vi "3D-10点建面算高度.vi"(9 "布尔":bool, 10 "Max 位置数组":cluster{"列":dbl, "行":dbl, "Z":dbl}[](array[cluster]), 11 "基准点数组":cluster{"列":dbl, "行":dbl, "Z":dbl}[](array[cluster])) -> (0 "Z":string[](array[string]), 1 "Result":string, 3 "Z轴相对高度":dbl[](array[numeric])=[0.07904724866187265, 0.12091362208012832, 0.13921122232312513, 0.04880031245592914, 1.3322676295365137e-15, 0.021807097148537454, 1.9984014443047706e-15, 0.020027978783221875, 0.014032416135081075, -0.06192666880740527, -0.09122658763869643, -3.663735981225413e-15])   [LabVIEW 2015]
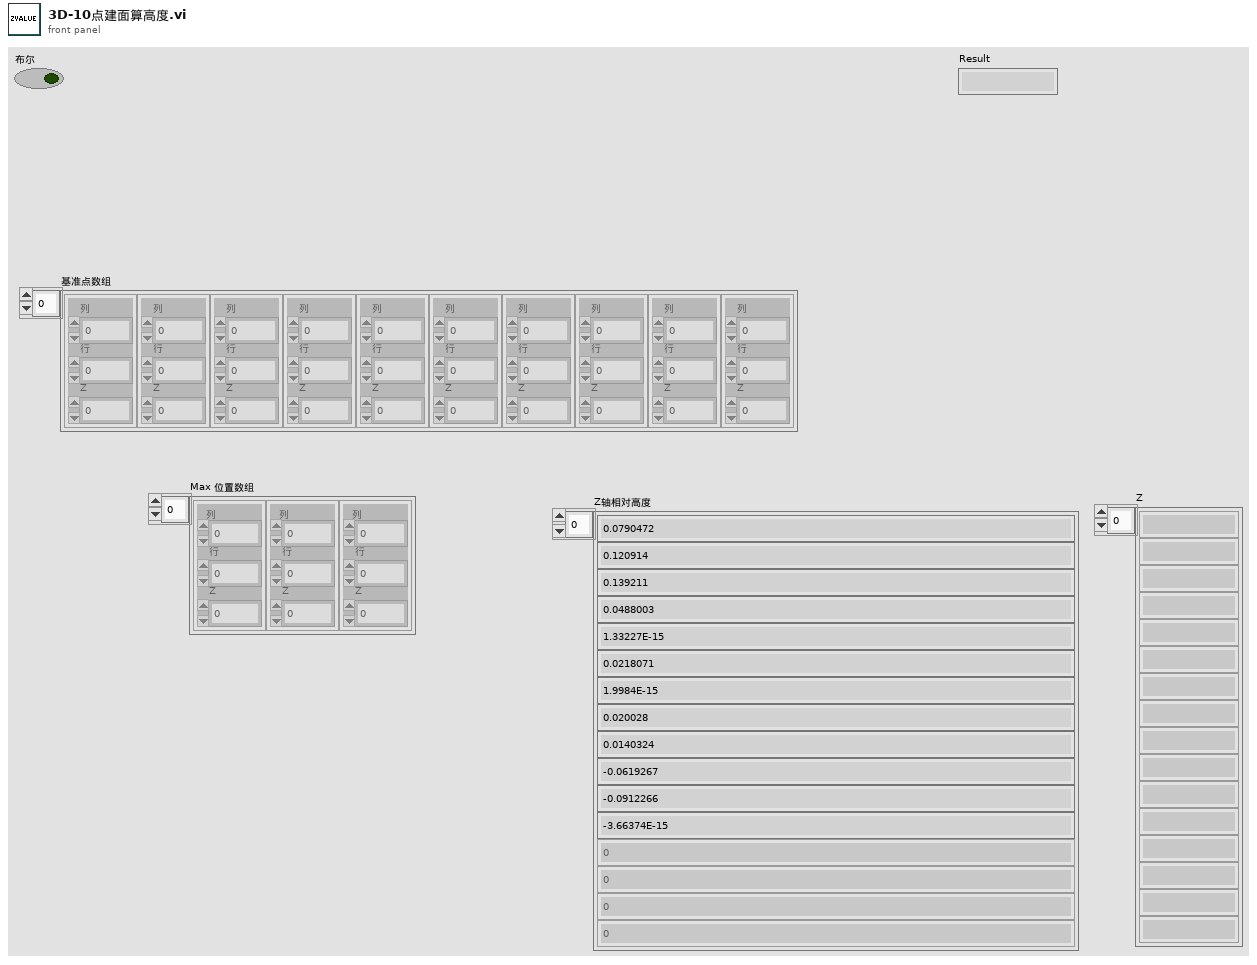
[diagram p1: front panel]
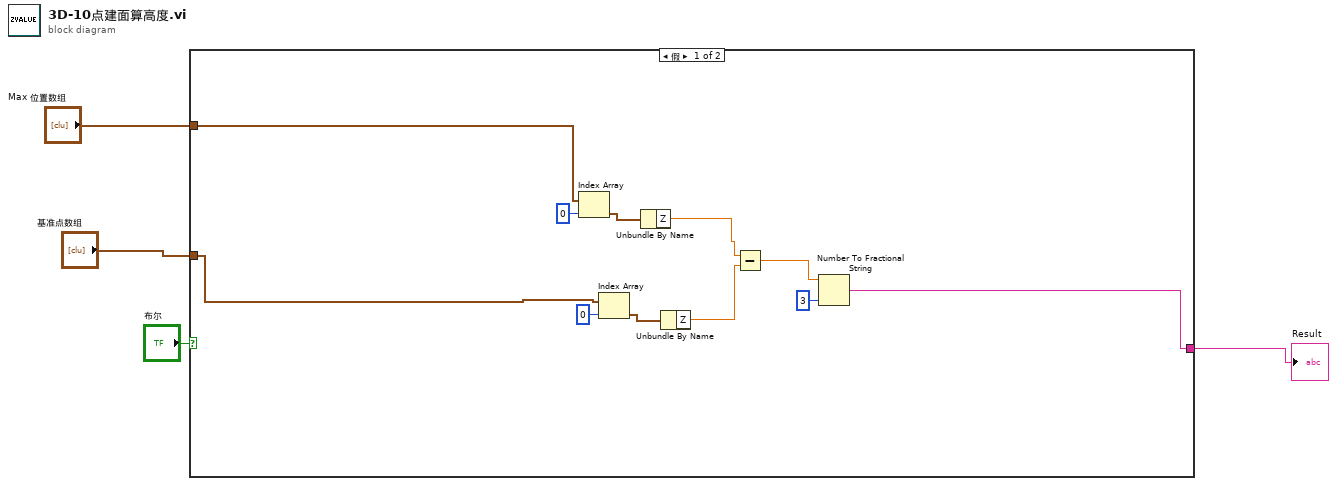
[diagram p0: block diagram]
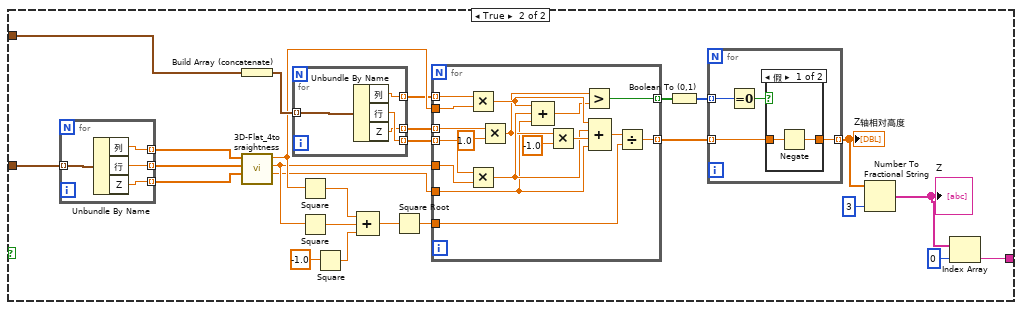
[diagram p2: hidden frame]
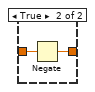
[diagram p3: hidden frame]
diagram:
  n1 = case shown="假" "布尔" {
    tunnel: "基准点数组" -> [w8 w41]
    tunnel: "Max 位置数组" -> [w9 w40]
    tunnel: [w7 w16] -> w1
    frame False {
      n2 = Index Array(array=w9, index=0 ("索引")) -> (element=w14:cluster{"列":dbl, "行":dbl, "Z":dbl})
      n3 = Index Array(array=w8, index=0 ("索引")) -> (element=w13:cluster{"列":dbl, "行":dbl, "Z":dbl})
      n4 = Unbundle By Name(w14) -> ("Z"=w6:dbl)
      n5 = Unbundle By Name(w13) -> ("Z"=w11:dbl)
      n6 = Subtract(x=w6, y=w11) -> (x-y=w5:dbl)
      n7 = Number To Fractional String(number=w5, precision (6)=i16 3 ("精度(6)")) -> (F-format string=w7:string)  [unwired: 2 in]
    }
    frame True {
      n8 = for {
        tunnel: w41 -> [w74] mode=indexing
        tunnel: [w73] -> w31 mode=indexing
        tunnel: [w72] -> w30 mode=indexing
        tunnel: [w71] -> w29 mode=indexing
        n9 = Unbundle By Name(w74) -> ("列"=w73:dbl, "行"=w72:dbl, "Z"=w71:dbl)
      }
      n10 = Build Array (concatenate)(w40) -> (w37:cluster{"列":dbl, "行":dbl, "Z":dbl}[])
      n11 = call "3D-Flat_4to sraightness.vi"("Z"=w29, "Y"=w30, "X"=w31) -> ("C"=w23:dbl, "B"=w24:dbl, "A"=w25:dbl)  [unwired: 4 in, 2 out]
      n12 = for {
        tunnel: w37 -> [w70] mode=indexing
        tunnel: [w69] -> w21 mode=indexing
        tunnel: [w68] -> w20 mode=indexing
        tunnel: [w67] -> w19 mode=indexing
        n13 = Unbundle By Name(w70) -> ("列"=w69:dbl, "行"=w68:dbl, "Z"=w67:dbl)
      }
      n14 = Square(x=w25) -> (x^2=w32:dbl)
      n15 = Square(x=w24) -> (x^2=w33:dbl)
      n16 = Square(x=-1.0) -> (x^2=w35:dbl)
      n17 = Compound Arithmetic op=ADD(w32, w33, w35) -> (w36:dbl)
      n18 = Square Root(x=w36) -> (sqrt(x)=w22:dbl)
      n19 = for {
        tunnel: w20 -> [w55] mode=indexing
        tunnel: w19 -> [w54] mode=indexing
        tunnel: [w58] -> w26 mode=indexing
        tunnel: [w57] -> w28 mode=indexing
        tunnel: w21 -> [w56] mode=indexing
        tunnel: w25 -> [w53]
        tunnel: w24 -> [w52]
        tunnel: w23 -> [w51]
        tunnel: w22 -> [w50]
        n20 = Multiply(x=w56, y=w53) -> (x*y=w63:dbl)
        n21 = Multiply(x=w55, y=w52) -> (x*y=w62:dbl)
        n22 = Multiply(x=w54, y=1.0) -> (x*y=w61:dbl)
        n23 = Compound Arithmetic op=ADD(w63, w62, w51) -> (w60:dbl)
        n24 = Multiply(x=w61, y=-1.0) -> (x*y=w64:dbl)
        n25 = Greater?(x=w61, y=w60) -> (0:w58:bool)
        n26 = Compound Arithmetic op=ADD(w63, w62, w64, w51) -> (w59:dbl)
        n27 = Divide(x=w59, y=w50) -> (x/y=w57:dbl)
      }
      n28 = Boolean To (0,1)(Boolean=w26) -> (0, 1=w27:i16[])
      n29 = for {
        tunnel: w28 -> [w43] mode=indexing
        tunnel: w27 -> [w45] mode=indexing
        tunnel: [w42] -> w18 mode=indexing
        n30 = Equal To 0?(x=w45) -> (x = 0?=w44:bool)
        n31 = case shown="假" w44 {
          tunnel: w43 -> [w46 w49]
          tunnel: [w47 w48] -> w42
          frame False {
            n32 = Negate(x=w46) -> (-x=w47:dbl)
          }
          frame True {
            n33 = Negate(x=w49) -> (-x=w48:dbl)
          }
        }
      }
      "Z轴相对高度" <- w18
      n34 = Number To Fractional String(number=w18, precision (6)=i16 3 ("精度(6)")) -> (F-format string=w39:string[])  [unwired: 2 in]
      "Z" <- w39
      n35 = Index Array(array=w39, index=0 ("索引")) -> (element=w16:string)
    }
  }
  "Result" <- w1
